vi "TimeInterpDouble_New.vi"(11 "MaxTime":dbl=1.0) -> (3 "TimeInterpDouble":T1)   [LabVIEW 2019, in "Trajectory_Library.lvlib"]
doc: "Create the data cluster for a TIME_INTERPOLATABLE_DOUBLE.\n\nThe TimeInterpolatableBuffer provides an easy way to estimate past measurements. One application might be in conjunction with the DifferentialDrivePoseEstimator, where knowledge of the robot pose at the time when vision or other global measurement were recorded is necessary, or for recording the past angles of mechanisms as measured by encoders.\n\nThe TIME_INTERPOLATABLE_DOUBLE stores and returns DOUBLE values.\n\nInputs:\n - Max Time -- The maximum time (seconds) of data to store in the buffer.\n\nOutputs:\n - Time Inter Double -- Created data structure cluster"
uses:
  TIME_INTERPOLATABLE_DOUBLE.ctl
  Trajectory_Library.lvlib
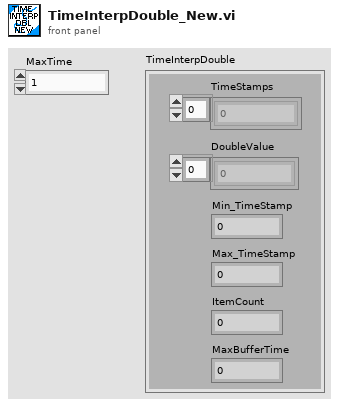
[diagram p1: front panel]
types:
  T1 = typedef "Trajectory_Library.lvlib/TIME_INTERPOLATABLE_DOUBLE.ctl" = cluster{"TimeStamps":dbl[], "DoubleValue":dbl[], "Min_TimeStamp":dbl, "Max_TimeStamp":dbl, "ItemCount":i32, "MaxBufferTime":dbl}
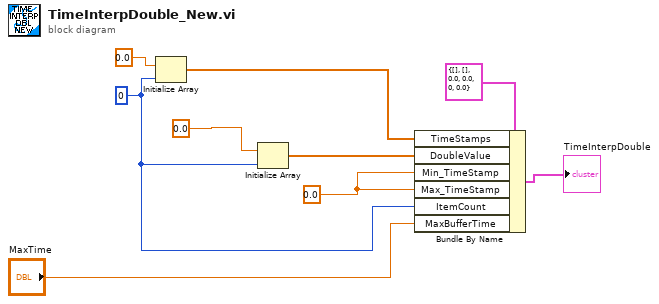
[diagram p0: block diagram]
diagram:
  w6 = 0.0 ("X")
  w3 = 0 ("dimension size")
  n1 = Initialize Array(0.0 ("element"), w3) -> (w7:dbl[])
  n2 = Initialize Array(0.0 ("element"), w3) -> (w4:dbl[])
  n3 = Bundle By Name(cluster=T1 {"TimeStamps"=[], "DoubleValue"=[], "Min_TimeStamp"=0.0, "Max_TimeStamp"=0.0, "ItemCount"=0, "MaxBufferTime"=0.0} ("TIME_INTERPOLATABLE_DOUBLE"), "TimeStamps"=w7, "DoubleValue"=w4, "Min_TimeStamp"=w6, "Max_TimeStamp"=w6, "ItemCount"=w3, "MaxBufferTime"="MaxTime") -> (→"TimeInterpDouble":T1)
